vi "save_scan.vi"(8 "error in":errorcluster, 10 "values in":dbl[](array[numeric])=[644.3, 644.3019999999999, 644.3039999999999, 644.3059999999998, 644.3079999999998, 644.3099999999997, 644.3119999999997, 644.3139999999996, 644.3159999999996, 644.3179999999995, 644.3199999999995, 644.3219999999994, 644.3239999999994, 644.3259999999993, 644.3279999999993, 644.3299999999992, 644.3319999999992, 644.3339999999992, 644.3359999999991, 644.337999999999, 644.339999999999, 644.341999999999, 644.3439999999989, 644.3459999999989, 644.3479999999988, 644.3499999999988, 644.3519999999987, 644.3539999999987, 644.3559999999986, 644.3579999999986, 644.3599999999985, 644.3619999999985, 644.3639999999984, 644.3659999999984, 644.3679999999983, 644.3699999999983, 644.3719999999983, 644.3739999999982, 644.3759999999982, 644.3779999999981, 644.3799999999981, 644.381999999998, 644.383999999998, 644.3859999999979, 644.3879999999979, 644.3899999999978, 644.3919999999978, 644.3939999999977, 644.3959999999977, 644.3979999999976, 644.3999999999976, 644.4019999999975, 644.4039999999975, 644.4059999999974, 644.4079999999974, 644.4099999999974, 644.4119999999973, 644.4139999999973, 644.4159999999972, 644.4179999999972, 644.4199999999971, 644.4219999999971, 644.423999999997, 644.425999999997, 644.4279999999969, 644.4299999999969, 644.4319999999968, 644.4339999999968, 644.4359999999967, 644.4379999999967, 644.4399999999966, 644.4419999999966, 644.4439999999965, 644.4459999999965, 644.4479999999965, 644.4499999999964, 644.4519999999964, 644.4539999999963, 644.4559999999963, 644.4579999999962, 644.4599999999962, 644.4619999999961, 644.4639999999961, 644.465999999996, 644.467999999996, 644.4699999999959, 644.4719999999959, 644.4739999999958, 644.4759999999958, 644.4779999999957, 644.4799999999957, 644.4819999999957, 644.4839999999956, 644.4859999999956, 644.4879999999955, 644.4899999999955, 644.4919999999954, 644.4939999999954, 644.4959999999953, 644.4979999999953, 644.4999999999952, 644.5019999999952, 644.5039999999951, 644.5059999999951, 644.507999999995, 644.509999999995, 644.5119999999949, 644.5139999999949, 644.5159999999948, 644.5179999999948, 644.5199999999948, 644.5219999999947, 644.5239999999947, 644.5259999999946, 644.5279999999946, 644.5299999999945, 644.5319999999945, 644.5339999999944, 644.5359999999944, 644.5379999999943, 644.5399999999943, 644.5419999999942, 644.5439999999942, 644.5459999999941, 644.5479999999941, 644.549999999994, 644.551999999994, 644.553999999994, 644.5559999999939, 644.5579999999939, 644.5599999999938, 644.5619999999938, 644.5639999999937, 644.5659999999937, 644.5679999999936, 644.5699999999936, 644.5719999999935, 644.5739999999935, 644.5759999999934, 644.5779999999934, 644.5799999999933, 644.5819999999933, 644.5839999999932, 644.5859999999932, 644.5879999999931, 644.5899999999931, 644.591999999993, 644.593999999993, 644.595999999993, 644.5979999999929, 644.5999999999929, 644.6019999999928, 644.6039999999928, 644.6059999999927, 644.6079999999927, 644.6099999999926, 644.6119999999926, 644.6139999999925, 644.6159999999925, 644.6179999999924, 644.6199999999924, 644.6219999999923, 644.6239999999923, 644.6259999999922, 644.6279999999922, 644.6299999999922, 644.6319999999921, 644.633999999992, 644.635999999992, 644.637999999992, 644.6399999999919, 644.6419999999919, 644.6439999999918, 644.6459999999918, 644.6479999999917, 644.6499999999917, 644.6519999999916, 644.6539999999916, 644.6559999999915, 644.6579999999915, 644.6599999999914, 644.6619999999914, 644.6639999999913, 644.6659999999913, 644.6679999999913, 644.6699999999912, 644.6719999999912, 644.6739999999911, 644.6759999999911, 644.677999999991, 644.679999999991, 644.6819999999909, 644.6839999999909, 644.6859999999908, 644.6879999999908, 644.6899999999907, 644.6919999999907, 644.6939999999906, 644.6959999999906, 644.6979999999905, 644.6999999999905] format="%#_8p", 11 "path":path caption="selected path") -> (0 "error out":errorcluster)   [LabVIEW 2017, in "tools.lvlib"]
uses:
  tools.lvlib
  <vilib>/Utility/file.llb/Write Delimited Spreadsheet (DBL).vi
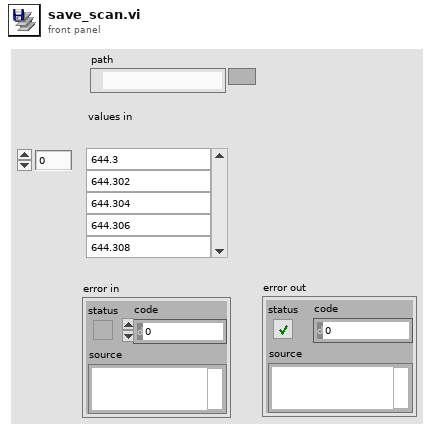
[diagram p1: front panel]
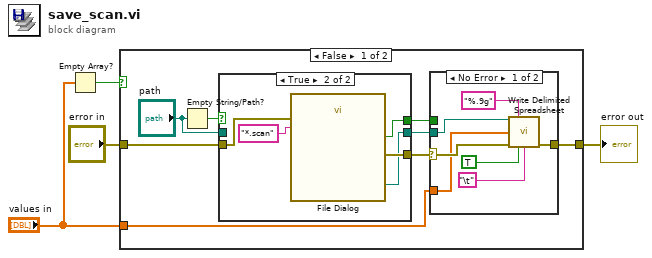
[diagram p0: block diagram]
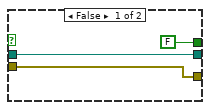
[diagram p2: hidden frame]
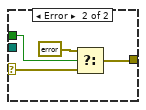
[diagram p3: hidden frame]
diagram:
  n1 = Empty Array?(array="values in") -> (empty?=w1:bool)
  n2 = case shown="False" w1 {
    tunnel: "error in" -> [w9 w32]
    tunnel: [w8 w32] -> w3
    tunnel: "values in" -> [w5 _]
    frame False {
      n3 = Empty String/Path?(string/path="path") -> (empty?=w7:bool)
      n4 = case shown="True" w7 {
        tunnel: [w14 w19] -> w12
        tunnel: [w15 w18] -> w11
        tunnel: [FALSE ("cancelled") w17] -> w10
        tunnel: w9 -> [w14 w16]
        tunnel: "path" -> [w15 _]
        frame False {
        }
        frame True {
          n5 = call "File Dialog"("error in"=w16, "pattern (all files)"="*.scan") -> ("selected path"=w18:path, "cancelled"=w17:bool, "error out"=w19:errorcluster)  [unwired: 10 in, 1 out]
        }
      }
      n6 = case shown="No Error" w12 {
        selector: w12 -> [w23 w31]
        tunnel: w11 -> [w25 _]
        tunnel: w5 -> [w21 _]
        tunnel: w10 -> [_ w29]
        tunnel: [w24 w28] -> w8
        frame No Error {
          n7 = call-poly <vilib>:"Write Delimited Spreadsheet.vi"("file path (dialog if empty)"=w25, "format (%.3f)"="%.9g", "1D data"=w21, "error in (no error)"=w23, "transpose? (no:F)"=TRUE, "delimiter (\\t)"="\t") -> ("error out"=w24:errorcluster)  [unwired: 8 in, 1 out]
        }
        frame Error {
          n8 = Select(t=errorcluster {"status"=FALSE, "code"=0, "source"=""}, s=w29, f=w31) -> (s? t:f=w28:errorcluster)
        }
      }
    }
    frame True {
    }
  }
  "error out" <- w3
